vi "Move From Output to Export Dir.vi"(0 "CL_G3_VIComponentBuilder.lvlib:Compound_Installer":refnum<class "Compound_Installer.lvclass">, 11 "error IO":errorcluster) -> (4 "CL_G3_VIComponentBuilder.lvlib:Compound_Installer":refnum<class "Compound_Installer.lvclass">, 15 "error out":errorcluster)   [LabVIEW 2017, in "CL_G3_VIComponentBuilder.lvlib" / "Compound_Installer.lvclass"]
doc: "The abstract implementation to match that of NI Spect export type."
uses:
  Compound_Installer.lvclass
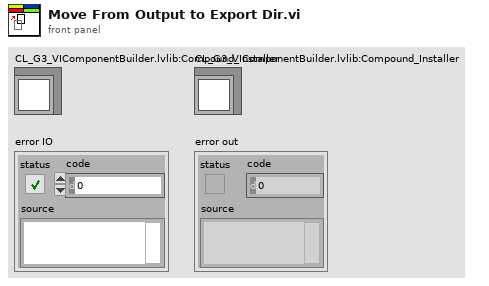
[diagram p1: front panel]
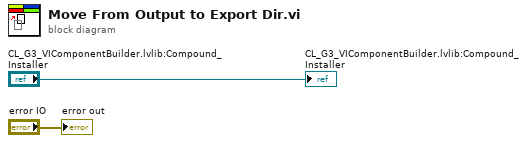
[diagram p0: block diagram]
diagram:
  "error out" <- "error IO"
  "CL_G3_VIComponentBuilder.lvlib:Compound_Installer" <- "CL_G3_VIComponentBuilder.lvlib:Compound_Installer"
